vi "Read Data Example.vi"() -> ()   [LabVIEW 2012, in "Digital Compass HMC5883L.lvlib"]
uses:
  Digital Compass HMC5883L.lvlib
  <vilib>/LabVIEW Interface for Arduino/LabVIEW Interface for Arduino.lvlib
panel:
  out "Y":i16
  out "Z":i16
  out "X":i16
  in  "stop":bool
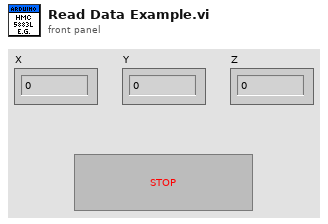
[diagram p1: front panel]
types:
  T1 = typedef "LabVIEW Interface for Arduino.lvlib/Arduino Resource.ctl" = cluster{"VISA resource":refnum<visa-resource-name>, "Board Type":T2, "Connection Type":enum8{"USB / Serial"}, "Bytes Per Packet (15)":u8}
  T2 = typedef "LabVIEW Interface for Arduino.lvlib/Board Type.ctl" = enum16{"Uno", "Dimuelanove w/Atmega 328", "Mega 2560"}
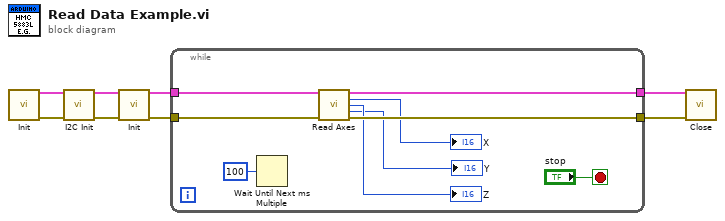
[diagram p0: block diagram]
diagram:
  n1 = call <vilib>:"Init.vi"() -> ("Arduino Resource"=w8:T1, "error out"=w5:errorcluster)  [unwired: 18 in]
  n2 = call <vilib>:"I2C Init.vi"("Arduino Resource"=w8, "error in"=w5) -> ("Arduino Resource"=w7:T1, "error out"=w6:errorcluster)  [unwired: 12 in]
  n3 = call <vilib>:"Init.vi"("Arduino Resource in"=w7, "error in (no error)"=w6) -> ("Arduino Resource Out"=w1:T1, "error out"=w4:errorcluster)  [unwired: 12 in]
  n4 = while {
    tunnel: w4 -> [w16]
    tunnel: [w15] -> w3
    tunnel: [w14] -> w2
    tunnel: w1 -> [w13]
    stop <- "stop" stop-if-true
    n5 = Wait Until Next ms Multiple(millisecond multiple=u32 100) -> ()  [unwired: 1 out]
    n6 = call "Read Axes.vi"("Arduino Resource"=w13, "error in (no error)"=w16) -> ("Arduino Resource"=w14:T1, "X"=→"X":i16, "Z"=→"Z":i16, "Y"=→"Y":i16, "error out"=w15:errorcluster)  [unwired: 9 in]
  }
  n7 = call <vilib>:"Close.vi"("Arduino Resource"=w2, "error in"=w3) -> ()  [unwired: 13 in, 1 out]
